vi "ActionVIOnDelete_RemoveSystemMappings_Parent.vi"(6 "All deleted Refs":T1[](array[typedef]) format="%.0x", 8 "error in (no error)":errorcluster, 11 "Item Ref in":T1 format="%.0x") -> (0 "error out":errorcluster, 3 "Item Ref out":T1 format="%.0x")   [LabVIEW 2016, in "LIN Frame Protection Addon System Explorer.lvlib"]
uses:
  LIN Frame Protection Addon System Explorer.lvlib
  <vilib>/NI Veristand/Custom Device API/Custom Device Item Ref.ctl
  Shared/LIN Frame Protection Addon Shared.lvlib
  <vilib>/NI Veristand/Custom Device API/Custom Device API.lvlib
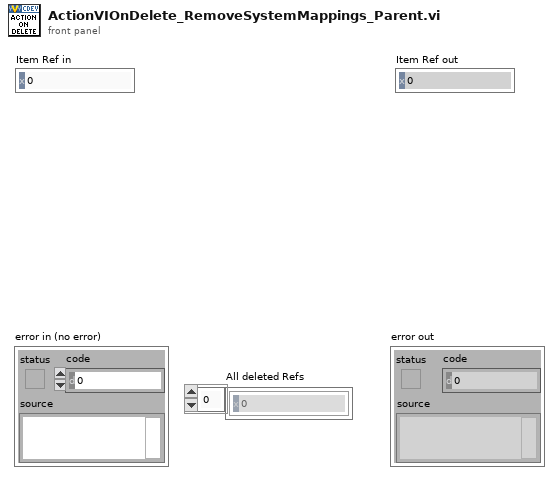
[diagram p1: front panel]
types:
  T1 = typedef "Custom Device API.lvlib/Custom Device Item Ref.ctl" = u64
  T2 = typedef "LIN Frame Protection Addon Shared.lvlib/FrameConfiguration.ctl" = cluster{"Input Channels":T3[], "Schedule_SumOfDelays":dbl, "Rolling Counter Count":dbl, "PCL Count":u64, "Max Count":dbl, "Frame ID":u32, "Rolling Counter":T3, "CRC":T3, "Frame Name":string, "Cluster":string, "Database":string, "Protection Type":T4}
  T3 = typedef "LIN Frame Protection Addon Shared.lvlib/InputChannelConfiguration.ctl" = cluster{"Start Bit":i32, "Name":string, "Node Path":string, "Number of bits":i32, "Scale":dbl, "Offset":dbl, "Data Type":u32}
  T4 = typedef "LIN Frame Protection Addon Shared.lvlib/Protection Type.ctl" = enum16{"Checksum", "CRC", "None (Counter Only)"}
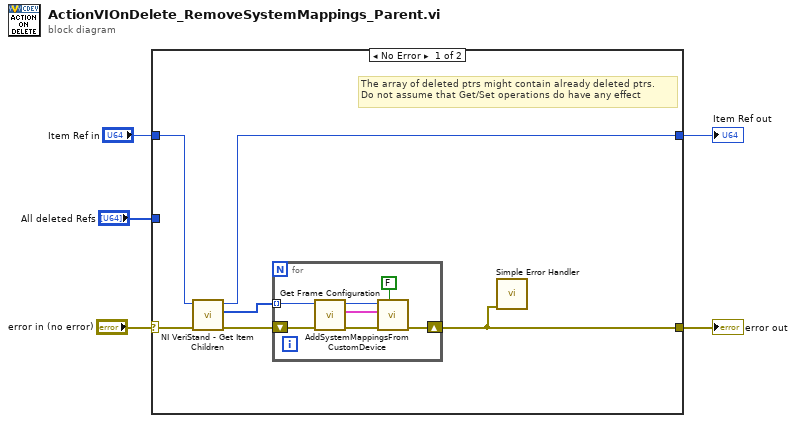
[diagram p0: block diagram]
diagram:
  n1 = case shown="No Error" "error in (no error)" {
    selector: "error in (no error)" -> [w10 w20]
    tunnel: [w11 w20] -> w4
    tunnel: "Item Ref in" -> [w8 w19]
    tunnel: [w7 w19] -> w2
    tunnel: "All deleted Refs" -> [_ _]
    frame No Error {
      # "The array of deleted ptrs might contain already deleted ptrs.\nDo not assume that Get/Set operations do have any effect"
      n2 = call <vilib>:"NI VeriStand - Get Item Children.vi"("error in (no error)"=w10, "Item Ref in"=w8) -> ("error out"=w9:errorcluster, "Child Refs"=w6:T1[], "Item Ref out"=w7:T1)  [unwired: 6 in, 1 out]
      n3 = for {
        shift-right: [w13] -> w11
        shift-left: w9 -> [w17]
        tunnel: w6 -> [w12] mode=indexing
        n4 = call "Get Frame Configuration.vi"("error in"=w17, "Parent Ref"=w12) -> ("error out"=w14:errorcluster, "Selected Channels"=w16:T2, "Parent Ref Out"=w15:T1)  [unwired: 7 in]
        n5 = call "AddSystemMappingsFromCustomDevice.vi"("Add? (T)"=FALSE, "error in"=w14, "Frame Configuration"=w16, "Node Ptr"=w15) -> ("error out"=w13:errorcluster)  [unwired: 5 in, 2 out]
      }
      n6 = call <vilib>:"Simple Error Handler.vi"("error in (no error)"=w11) -> ()  [unwired: 4 in, 5 out]
    }
    frame Error {
    }
  }
  "error out" <- w4
  "Item Ref out" <- w2
